vi "Calculations.vi"(0 "Trial in Progress IN":bool, 1 "DIO":bool[](array[boolean]), 2 "Trial Number":i16, 3 "cam_vel_ai_vlt":sgl[](array[numeric]), 5 "Sample Rate(s)":dbl=0.002 format="%.3f", 9 "Time Into Trial IN":dbl, 11 "Trial In Progress IN":T1, 12 "Inter-Trial Interval IN":bool) -> (4 "Data Cluster OUT":T2 {"Seconds Into Trial(s)" format="%#.10g"}, 6 "Trial Fraction of 1 Reached?":bool, 8 "Timeout Due to Mouse Not Moving?":bool, 10 "Wall MM Outputs":sgl[](array[numeric]), 14 "Trial Fraction OUT":dbl, 15 "Inter-Trial Interval Complete?":bool)   [LabVIEW 2018]
uses:
  controls/Data To Save.ctl
  controls/Trial Config Settings.ctl
  <vilib>/ptbypt/NI_PtbyPt.lvlib
  controls/RT_Cluster.ctl
panel:
  out "Speed_Time_Length":i32
  out "mean_lat_vel":dbl
  out "mean_for_vel":dbl
  out "Vball":dbl format="%.3f"
  out "lat_vel_array":dbl[](array[numeric])
  out "for_vel_array":dbl[](array[numeric])
  out "Cur_Speed_Ind":i32
  out "A_calib_matrix_row1":dbl[](array[numeric])
  out "A_calib_matrix_row0":dbl[](array[numeric])
  out "lat_ball_motion":dbl
  out "for_ball_motion":dbl
  out "zero_V":dbl[](array[numeric])
  out "step_V":dbl
  out "cam_vel_steps":dbl[](array[numeric])
  # "aClck_DI\nframe_clock_DO\nwhisker_video_ctrl_DO\nlick_signal_DI\nwater_valve_trigger\nlaser_ctrl\nleft_texture_ctrl_DO\nright_texture_ctrl_DO\ntrial_ephys_ctrl_DO\ntrial_iti_ctrl_DO\ntrial_on_ctrl_DO\nephys_clock_DO"
  # "*If Speed_Time_Length = 250\nthen averages are calculated every\n0.5 seconds since 1 data save takes\nplace every 0.002 seconds."
  # "="
  # "="
  # "avg"
  # "mean_for_vel"
  # "for_ball_motion (speed_time_length)"
  # "="
  # "="
  # "avg"
  # "mean_lat_vel"
  # "lat_ball_motion (speed_time_length)"
  # "cm/s"
  # "cm/s"
  # "2"
  # "2"
  # "="
  # "+"
  # "cm/s"
  # "for_ball_motion"
  # "lat_ball_motion"
  # "Left Wall"
  # "Vdc"
  # "Right Wall"
  # "Vdc"
  # "A_calib(0,0) x cam_vel_steps(0)"
  # "="
  # "A_calib(0,1) x cam_vel_steps(1)"
  # "sum"
  # "cm/s"
  # "A_calib(0,2) x cam_vel_steps(2)"
  # "A_calib(0,3) x cam_vel_steps(3)"
  # "A_calib(1,0) x cam_vel_steps(0)"
  # "="
  # "A_calib(1,1) x cam_vel_steps(1)"
  # "sum"
  # "cm/s"
  # "A_calib(1,2) x cam_vel_steps(2)"
  # "A_calib(1,3) x cam_vel_steps(3)"
  # "minus"
  # "="
  # "round"
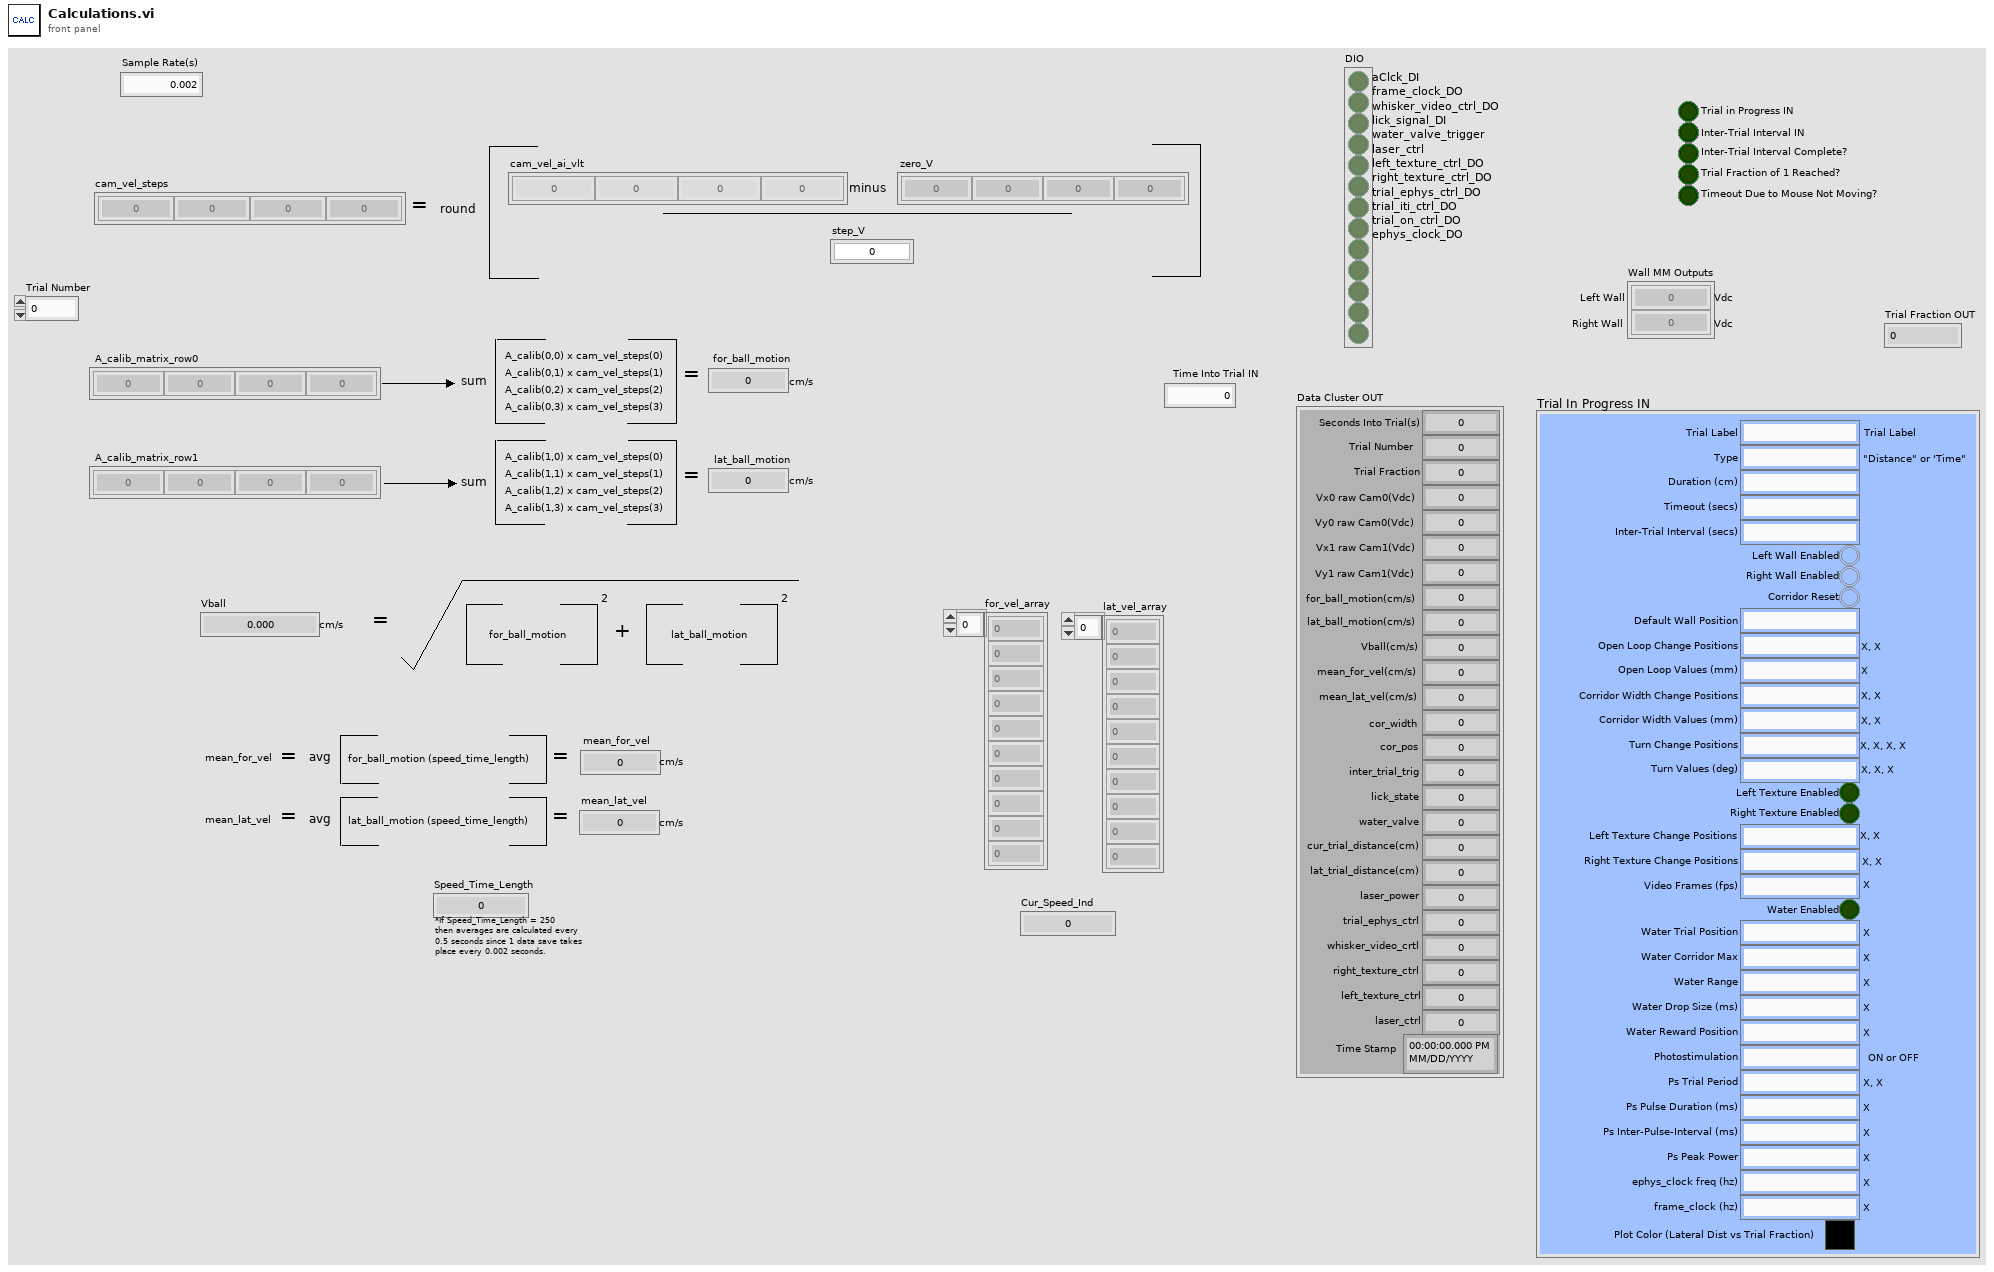
[diagram p1: front panel]
types:
  T1 = typedef "Trial Config Settings.ctl" = cluster{"Trial Label":string, "Type":string, "Timeout (secs)":string, "Inter-Trial Interval (secs)":string, "Left Wall Enabled":bool, "Right Wall Enabled":bool, "Corridor Reset":bool, "Default Wall Position":string, "Open Loop Change Positions":string, "Open Loop Values (mm)":string, "Corridor Width Change Positions":string, "Corridor Width Values (mm) ":string, "Turn Change Positions":string, "Turn Values (deg)":string, "Left Texture Change Positions":string, "Right Texture Change Positions":string, "Video Frames (fps)":string, "Water Enabled":bool, "Water Trial Position":string, "Photostimulation":string, "Water Corridor Max":string, "Water Range":string, "Water Drop Size (ms)":string, "Water Reward Position":string, "Duration (cm)":string, "Left Texture Enabled":bool, "Right Texture Enabled":bool, "Ps Trial Period":string, "Ps Inter-Pulse-Interval (ms)":string, "Ps Peak Power":string, "Ps Pulse Duration (ms)":string, "ephys_clock freq (hz)":string, "frame_clock (hz)":string, "Plot Color (Lateral Dist vs Trial Fraction)":u32}
  T2 = typedef "Data To Save.ctl" = cluster{"Vx0 raw Cam0(Vdc)":sgl, "Vy0 raw Cam0(Vdc)":sgl, "Vx1 raw Cam1(Vdc)":sgl, "Vy1 raw Cam1(Vdc)":sgl, "Seconds Into Trial(s)":dbl, "cor_width":sgl, "cor_pos":sgl, "for_ball_motion(cm/s)":sgl, "lat_ball_motion(cm/s)":sgl, "Vball(cm/s)":sgl, "mean_for_vel(cm/s)":sgl, "mean_lat_vel(cm/s)":sgl, "Trial Fraction":dbl, "Trial Number":i16, "inter_trial_trig":i16, "lick_state":i16, "water_valve":i16, "cur_trial_distance(cm)":dbl, "lat_trial_distance(cm)":dbl, "laser_power":dbl, "trial_ephys_ctrl":i16, "whisker_video_crtl":i16, "right_texture_ctrl":i16, "left_texture_ctrl":i16, "laser_ctrl":i16, "Time Stamp":timestamp}
  T3 = typedef "RT_Cluster.ctl" = cluster{"Data Cluster OUT":T2, "Corridor Reset":bool, "Wall Analog Outputs":sgl[], "Trial Fraction of 1 Reached?":bool, "Timeout Due to Mouse Not Moving?":bool, "Inter-Trial Interval Complete?":bool, "appended array":dbl[], "appended array 2":dbl[]}
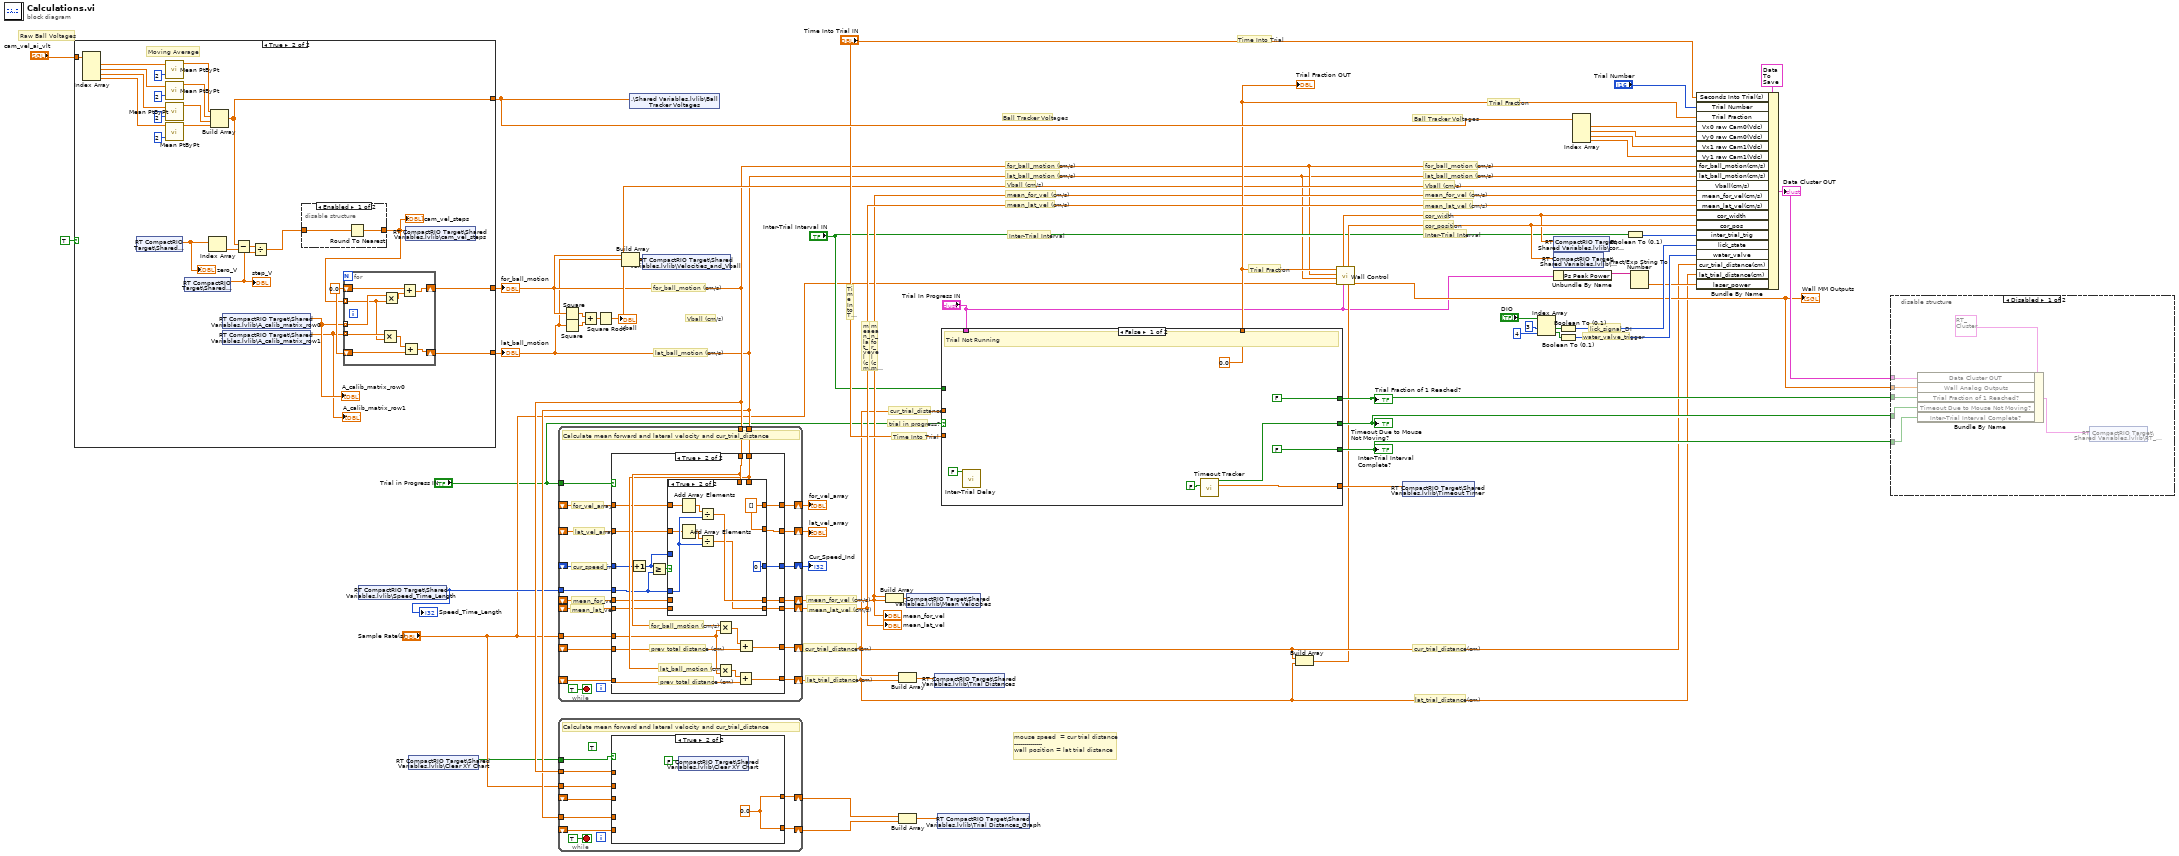
[diagram p0: block diagram]
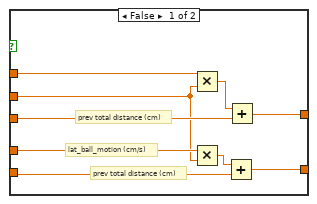
[diagram p3: hidden frame]
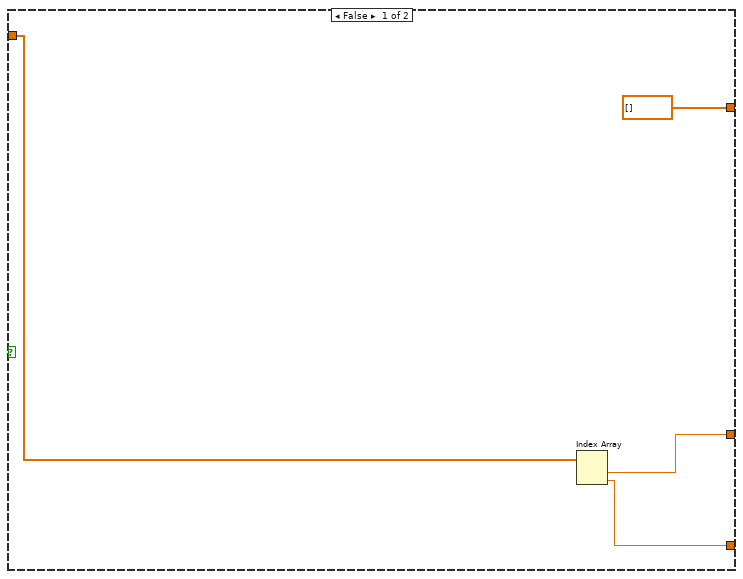
[diagram p4: hidden frame]
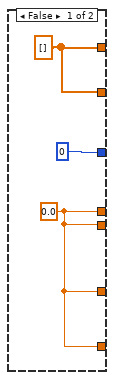
[diagram p6: hidden frame]
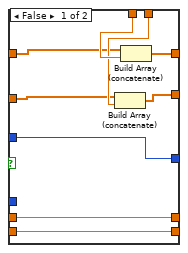
[diagram p7: hidden frame]
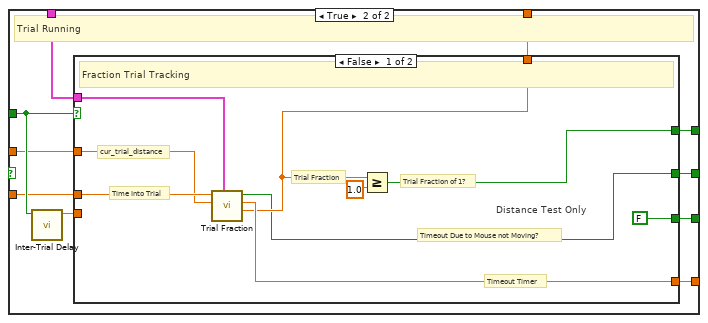
[diagram p8: hidden frame]
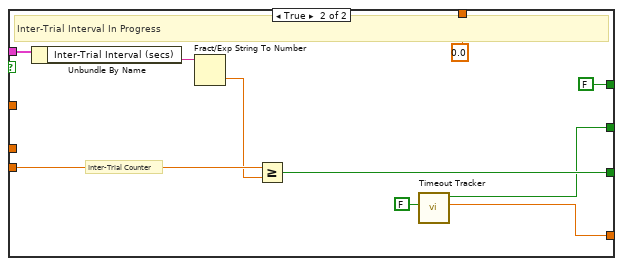
[diagram p9: hidden frame]
diagram:
  # "mouse speed  = cur trial distance\n--------------\nwall position = lat trial distance"
  # "Trial Fraction"
  # "lat_trial_distance(cm)"
  # "mean_for_vel (cm/s)"
  # "mean_lat_vel (cm/s)"
  # "cur_trial_distance(cm)"
  # "trial in progress?"
  # "for_ball_motion (cm/s)"
  # "lat_ball_motion (cm/s)"
  # "mean_lat_vel (cm/s)"
  # "mean_for_vel (cm/s)"
  # "Vball (cm/s)"
  # "lat_trial_distance(cm)"
  # "Inter-Trial Interval"
  # "cur_trial_distance(cm)"
  # "mean_for_vel (cm/s)"
  # "mean_lat_vel (cm/s)"
  # "Time Into Trial"
  # "Time Into Trial"
  # "cur_trial_distance"
  # "Vball (cm/s)"
  # "for_ball_motion (cm/s)"
  # "lat_ball_motion (cm/s)"
  # "Inter-Trial Interval"
  # "cor_position"
  # "cor_width"
  # "Ball Tracker Voltages"
  # "Time Into Trial"
  # "Ball Tracker Voltages"
  # "for_ball_motion (cm/s)"
  # "lat_ball_motion (cm/s)"
  # "mean_lat_vel (cm/s)"
  # "mean_for_vel (cm/s)"
  # "Vball (cm/s)"
  # "Trial Fraction"
  # "water_valve_trigger"
  # "lick_signal_DI"
  # "Raw Ball Voltages"
  n1 = case shown="True" TRUE {
    tunnel: "cam_vel_ai_vlt" -> [w59 w69]
    tunnel: [dbl[] [] w64] -> w48
    tunnel: [w58 w61] -> w13
    tunnel: [w57 w60] -> w12
    frame False {
      n2 = Index Array(array=w59) -> (element #1=w58:sgl, element #2=w57:sgl)  [unwired: 2 in]
    }
    frame True {
      w84 = 0.0
      # "Moving Average"
      n3 = Index Array(array=w69) -> (element #1=w68:sgl, element #2=w67:sgl, element #3=w66:sgl, element #4=w65:sgl)  [unwired: 4 in]
      n4 = shared-variable "RT CompactRIO Target\\Shared Variables.lvlib\\zero_V"() -> (w80:dbl[])  [unwired: 1 in, 1 out]
      "zero_V" <- w80
      n5 = call <vilib>:"Mean PtByPt.vi"("x"=w68, "sample length"=2) -> ("mean"=w63:dbl)  [unwired: 2 in, 1 out]
      n6 = call <vilib>:"Mean PtByPt.vi"("x"=w67, "sample length"=2) -> ("mean"=w72:dbl)  [unwired: 2 in, 1 out]
      n7 = call <vilib>:"Mean PtByPt.vi"("x"=w66, "sample length"=2) -> ("mean"=w71:dbl)  [unwired: 2 in, 1 out]
      n8 = call <vilib>:"Mean PtByPt.vi"("x"=w65, "sample length"=2) -> ("mean"=w70:dbl)  [unwired: 2 in, 1 out]
      n9 = shared-variable "RT CompactRIO Target\\Shared Variables.lvlib\\step_V"() -> (w79:dbl)  [unwired: 1 in, 1 out]
      "step_V" <- w79
      n10 = Index Array(array=w80) -> (element=w82:dbl)  [unwired: 1 in]
      n11 = Build Array(w63, w72, w71, w70) -> (w64:dbl[])
      n12 = shared-variable "RT CompactRIO Target\\Shared Variables.lvlib\\A_calib_matrix_row0"() -> (w78:dbl[])  [unwired: 1 in, 1 out]
      "A_calib_matrix_row0" <- w78
      n13 = shared-variable "RT CompactRIO Target\\Shared Variables.lvlib\\A_calib_matrix_row1"() -> (w77:dbl[])  [unwired: 1 in, 1 out]
      "A_calib_matrix_row1" <- w77
      n14 = Subtract ("Subtract.vi")(x=w64, y=w82) -> (x-y=w83:dbl[])
      n15 = Divide(x=w83, y=w79) -> (x/y=w81:dbl[])
      n16 = disable-structure shown="Enabled" {
        disable-tunnel: w81 -> [w86 w87]
        disable-tunnel: [w85 w87] -> w62
        frame Enabled {
          n17 = Round To Nearest(number=w86) -> (nearest integer value=w85:dbl[])
        }
        frame Disabled {
        }
      }
      "cam_vel_steps" <- w62
      n18 = for {
        tunnel: w78 -> [w96] mode=indexing
        tunnel: w77 -> [w95] mode=indexing
        tunnel: w62 -> [w94] mode=indexing
        shift-right: [w91] -> w61
        shift-left: w84 -> [w92]
        shift-right: [w90] -> w60
        shift-left: w84 -> [w88]
        n19 = Multiply(x=w95, y=w94) -> (x*y=w89:dbl)
        n20 = Multiply(x=w96, y=w94) -> (x*y=w93:dbl)
        n21 = Add(x=w92, y=w93) -> (x+y=w91:dbl)
        n22 = Add(x=w89, y=w88) -> (x+y=w90:dbl)
      }
      n23 = shared-variable "RT CompactRIO Target\\Shared Variables.lvlib\\cam_vel_steps"(w62) -> ()  [unwired: 1 in, 1 out]
    }
  }
  "for_ball_motion" <- w13
  "lat_ball_motion" <- w12
  n24 = shared-variable "RT CompactRIO Target\\Shared Variables.lvlib\\Speed_Time_Length"() -> (w11:i32)  [unwired: 1 in, 1 out]
  "Speed_Time_Length" <- w11
  n25 = shared-variable "RT CompactRIO Target\\Shared Variables.lvlib\\Clear XY Chart"() -> (w2:bool)  [unwired: 1 in, 1 out]
  n26 = while {
    tunnel: w13 -> [w116]
    tunnel: w12 -> [w115]
    shift-right: [w114] -> w25
    shift-left: _ -> [w111]
    shift-right: [w113] -> w24
    shift-left: _ -> [w110]
    shift-right: [w108] -> w23
    shift-left: _ -> [w109]
    shift-right: [w106] -> w50
    shift-left: _ -> [w104]
    shift-right: [w107] -> w28
    shift-left: _ -> [w105]
    tunnel: w11 -> [w103]
    tunnel: "Trial in Progress IN" -> [w98]
    shift-right: [w102] -> w6
    shift-left: _ -> [w101]
    shift-right: [w100] -> w5
    shift-left: _ -> [w99]
    tunnel: "Sample Rate(s)" -> [w97]
    stop <- TRUE stop-if-true
    # "mean_for_vel"
    # "mean_lat_vel"
    # "cur_speed_ind"
    # "lat_vel_array"
    # "for_vel_array"
    # "Calculate mean forward and lateral velocity and cur_trial_distance"
    n27 = case shown="True" w98 {
      tunnel: w116 -> [_ w141]
      tunnel: w115 -> [_ w140]
      tunnel: [w119 w139] -> w114
      tunnel: [w119 w138] -> w113
      tunnel: w111 -> [_ w137]
      tunnel: w110 -> [_ w136]
      tunnel: w109 -> [_ w135]
      tunnel: [0 w134] -> w108
      tunnel: [w117 w133] -> w107
      tunnel: [w117 w132] -> w106
      tunnel: w105 -> [_ w131]
      tunnel: w104 -> [_ w130]
      tunnel: w103 -> [_ w129]
      tunnel: [w117 w128] -> w102
      tunnel: w101 -> [_ w127]
      tunnel: [w117 w126] -> w100
      tunnel: w99 -> [_ w125]
      tunnel: w97 -> [_ w120]
      frame False {
        w119 = dbl[] []
        w117 = 0.0 ("mean_for_vel")
      }
      frame True {
        # "prev total distance (cm)"
        # "lat_ball_motion (cm/s)"
        # "prev total distance (cm)"
        # "for_ball_motion (cm/s)"
        n28 = Increment(x=w135) -> (x+1=w123:i32)
        n29 = Greater Or Equal?(x=w123, y=w129) -> (x >= y?=w124:bool)
        n30 = case shown="True" w124 {
          tunnel: [w149 w159] -> w139
          tunnel: [w147 w159] -> w138
          tunnel: w129 -> [_ w156]
          tunnel: w141 -> [w150 _]
          tunnel: w140 -> [w148 _]
          tunnel: w137 -> [w146 w155]
          tunnel: w136 -> [w145 w154]
          tunnel: [w144 0] -> w134
          tunnel: w123 -> [w144 _]
          tunnel: [w143 w152] -> w133
          tunnel: [w142 w151] -> w132
          tunnel: w131 -> [w143 _]
          tunnel: w130 -> [w142 _]
          frame False {
            n31 = Build Array (concatenate)(w145, w148) -> (w147:dbl[])
            n32 = Build Array (concatenate)(w146, w150) -> (w149:dbl[])
          }
          frame True {
            w159 = dbl[] []
            n33 = Add Array Elements(numeric array=w155) -> (sum=w158:dbl)
            n34 = Add Array Elements(numeric array=w154) -> (sum=w157:dbl)
            n35 = Divide(x=w158, y=w156) -> (x/y=w152:dbl)
            n36 = Divide(x=w157, y=w156) -> (x/y=w151:dbl)
          }
        }
        n37 = Multiply(x=w141, y=w120) -> (x*y=w122:dbl)
        n38 = Multiply(x=w140, y=w120) -> (x*y=w121:dbl)
        n39 = Add(x=w121, y=w125) -> (x+y=w126:dbl)
        n40 = Add(x=w122, y=w127) -> (x+y=w128:dbl)
      }
    }
  }
  "mean_for_vel" <- w28
  "mean_lat_vel" <- w50
  "for_vel_array" <- w25
  "lat_vel_array" <- w24
  "Cur_Speed_Ind" <- w23
  n41 = while {
    tunnel: w13 -> [w168]
    tunnel: w12 -> [w167]
    shift-right: [w165] -> w8
    shift-left: _ -> [w164]
    shift-right: [w163] -> w9
    shift-left: _ -> [w162]
    tunnel: "Sample Rate(s)" -> [w161]
    tunnel: w2 -> [w160]
    stop <- TRUE stop-if-true
    (unwired) TRUE
    # "Calculate mean forward and lateral velocity and cur_trial_distance"
    n42 = case shown="True" w160 {
      tunnel: w168 -> [w177 _]
      tunnel: w167 -> [w176 _]
      tunnel: [w175 w179] -> w165
      tunnel: w164 -> [w174 _]
      tunnel: [w173 w179] -> w163
      tunnel: w162 -> [w172 _]
      tunnel: w161 -> [w169 _]
      frame False {
        # "prev total distance (cm)"
        # "lat_ball_motion (cm/s)"
        # "prev total distance (cm)"
        n43 = Multiply(x=w177, y=w169) -> (x*y=w171:dbl)
        n44 = Multiply(x=w176, y=w169) -> (x*y=w170:dbl)
        n45 = Add(x=w170, y=w172) -> (x+y=w173:dbl)
        n46 = Add(x=w171, y=w174) -> (x+y=w175:dbl)
      }
      frame True {
        w179 = 0.0 ("mean_for_vel")
        n47 = shared-variable "RT CompactRIO Target\\Shared Variables.lvlib\\Clear XY Chart"(FALSE ("Clear XY Chart")) -> ()  [unwired: 1 in, 1 out]
      }
    }
  }
  n48 = Square(x=w13) -> (x^2=w31:dbl)
  n49 = Square(x=w12) -> (x^2=w30:dbl)
  n50 = Add(x=w31, y=w30) -> (x+y=w29:dbl)
  n51 = Square Root(x=w29) -> (sqrt(x)=w22:dbl)
  "Vball" <- w22
  n52 = Build Array(w13, w12, w22) -> (w54:dbl[])
  n53 = shared-variable ".\\Shared Variables.lvlib\\Ball Tracker Voltages"(w48) -> ()  [unwired: 1 in, 1 out]
  n54 = shared-variable "RT CompactRIO Target\\Shared Variables.lvlib\\Velocities_and_Vball"(w54) -> ()  [unwired: 1 in, 1 out]
  n55 = Build Array(w28, w28) -> (w55:dbl[])
  n56 = Build Array(w6, w5) -> (w21:dbl[])
  n57 = Build Array(w8, w9) -> (w7:dbl[])
  n58 = shared-variable "RT CompactRIO Target\\Shared Variables.lvlib\\Mean Velocities"(w55) -> ()  [unwired: 1 in, 1 out]
  n59 = shared-variable "RT CompactRIO Target\\Shared Variables.lvlib\\Trial Distances"(w21) -> ()  [unwired: 1 in, 1 out]
  n60 = shared-variable "RT CompactRIO Target\\Shared Variables.lvlib\\Trial Distances_Graph"(w7) -> ()  [unwired: 1 in, 1 out]
  n61 = case shown="False" "Trial in Progress IN" {
    tunnel: "Inter-Trial Interval IN" -> [_ w195]
    tunnel: "Trial In Progress IN" -> [_ w194]
    tunnel: "Time Into Trial IN" -> [_ w193]
    tunnel: w6 -> [_ w192]
    tunnel: [w185 w191] -> w34
    tunnel: [FALSE w190] -> w17
    tunnel: [FALSE w189] -> w19
    tunnel: [0.0 ("Trial Fraction") w188] -> w35
    tunnel: [w180 w187] -> w18
    frame False {
      # "Trial Not Running"
      n62 = call "Inter-Trial Delay.vi"("Start Inter-Trial Delay?"=FALSE) -> ()  [unwired: 10 in, 1 out]
      n63 = call "Timeout Tracker.vi"("Mouse Not Moving?"=FALSE) -> ("Timeout Timer"=w185:dbl, "Timeout"=w180:bool)  [unwired: 9 in]
    }
    frame True {
      # "Trial Running"
      n64 = call "Inter-Trial Delay.vi"("Start Inter-Trial Delay?"=w195) -> ("Inter-Trial Counter (secs)"=w196:dbl)  [unwired: 10 in]
      n65 = case shown="False" w195 {
        tunnel: [w202 w214] -> w191
        tunnel: w196 -> [_ w213]
        tunnel: w194 -> [w204 w212]
        tunnel: w193 -> [w203 _]
        tunnel: w192 -> [w197 _]
        tunnel: [FALSE w209] -> w190
        tunnel: [w199 FALSE] -> w189
        tunnel: [w200 0.0 ("Trial Fraction")] -> w188
        tunnel: [w198 w206] -> w187
        frame False {
          # "cur_trial_distance"
          # "Timeout Timer"
          # "Distance Test Only"
          # "Timeout Due to Mouse not Moving?"
          # "Time Into Trial"
          # "Trial Fraction of 1?"
          # "Trial Fraction"
          # "Fraction Trial Tracking"
          n66 = call "Trial Fraction.vi"("Trial In Progress IN"=w204, "cur_trial_dist"=w197, "Time into Trial"=w203) -> ("Trial Fraction"=w200:dbl, "Timeout Timer"=w202:dbl, "Timeout?"=w198:bool)  [unwired: 6 in]
          n67 = Greater Or Equal?(x=w200, y=1.0) -> (x >= y?=w199:bool)
        }
        frame True {
          # "Inter-Trial Counter"
          # "Inter-Trial Interval In Progress"
          n68 = Unbundle By Name(w212) -> ("Inter-Trial Interval (secs)"=w211:string)
          n69 = Fract/Exp String To Number(string=w211) -> (number=w210:dbl)  [unwired: 3 in, 1 out]
          n70 = Greater Or Equal?(x=w213, y=w210) -> (x >= y?=w209:bool)
          n71 = call "Timeout Tracker.vi"("Mouse Not Moving?"=FALSE) -> ("Timeout Timer"=w214:dbl, "Timeout"=w206:bool)  [unwired: 9 in]
        }
      }
    }
  }
  "Inter-Trial Interval Complete?" <- w17
  "Trial Fraction of 1 Reached?" <- w19
  "Trial Fraction OUT" <- w35
  "Timeout Due to Mouse Not Moving?" <- w18
  n72 = Build Array(w6, w5) -> (w4:dbl[])
  n73 = call "Wall Control.vi"("Trial Distances"=w4, "Trial In Progress IN"="Trial In Progress IN", "Sample Rate(s)"="Sample Rate(s)", "lat_ball_motion IN"=w12, "for_ball_motion IN"=w13, "Trial Fraction IN"=w35) -> ("Wall MM Outputs"=w15:dbl[], "cor_pos OUT"=w33:dbl, "cor_width OUT"=w32:dbl)  [unwired: 3 in]
  "Wall MM Outputs" <- w15
  n74 = shared-variable "RT CompactRIO Target\\Shared Variables.lvlib\\Timeout Timer"(w34) -> ()  [unwired: 1 in, 1 out]
  n75 = Index Array(array="DIO", index #1=3 ("index"), index #2=4 ("index")) -> (element #1=w43:bool, element #2=w38:bool)
  n76 = shared-variable "RT CompactRIO Target\\Shared Variables.lvlib\\cor_width"(w32) -> ()  [unwired: 1 in, 1 out]
  n77 = shared-variable "RT CompactRIO Target\\Shared Variables.lvlib\\cor_pos"(w33) -> ()  [unwired: 1 in, 1 out]
  n78 = Unbundle By Name("Trial In Progress IN") -> ("Ps Peak Power"=w27:string)
  n79 = Boolean To (0,1)(Boolean=w43) -> (0, 1=w42:i16)
  n80 = Boolean To (0,1)(Boolean=w38) -> (0, 1=w37:i16)
  n81 = Index Array(array=w48) -> (element #1=w46:dbl, element #2=w47:dbl, element #3=w52:dbl, element #4=w51:dbl)  [unwired: 4 in]
  n82 = Boolean To (0,1)(Boolean="Inter-Trial Interval IN") -> (0, 1=w40:i16)
  n83 = Fract/Exp String To Number(string=w27) -> (number=w26:dbl)  [unwired: 3 in, 1 out]
  n84 = Bundle By Name(cluster=T2 {"Vx0 raw Cam0(Vdc)"=0.0, "Vy0 raw Cam0(Vdc)"=0.0, "Vx1 raw Cam1(Vdc)"=0.0, "Vy1 raw Cam1(Vdc)"=0.0, "Seconds Into Trial(s)"=0.0, "cor_width"=0.0, "cor_pos"=0.0, "for_ball_motion(cm/s)"=0.0, "lat_ball_motion(cm/s)"=0.0, "Vball(cm/s)"=0.0, "mean_for_vel(cm/s)"=0.0, "mean_lat_vel(cm/s)"=0.0, "Trial Fraction"=0.0, "Trial Number"=0, "inter_trial_trig"=0, "lick_state"=0, "water_valve"=0, "cur_trial_distance(cm)"=0.0, "lat_trial_distance(cm)"=0.0, "laser_power"=0.0, "trial_ephys_ctrl"=0, "whisker_video_crtl"=0, "right_texture_ctrl"=0, "left_texture_ctrl"=0, "laser_ctrl"=0, "Time Stamp"=timestamp(0 s since 1904-01-01)} ("Data"), "Seconds Into Trial(s)"="Time Into Trial IN", "Trial Number"="Trial Number", "Trial Fraction"=w35, "Vx0 raw Cam0(Vdc)"=w46, "Vy0 raw Cam0(Vdc)"=w47, "Vx1 raw Cam1(Vdc)"=w52, "Vy1 raw Cam1(Vdc)"=w51, "for_ball_motion(cm/s)"=w13, "lat_ball_motion(cm/s)"=w12, "Vball(cm/s)"=w22, "mean_for_vel(cm/s)"=w28, "mean_lat_vel(cm/s)"=w50, "cor_width"=w32, "cor_pos"=w33, "inter_trial_trig"=w40, "lick_state"=w42, "water_valve"=w37, "cur_trial_distance(cm)"=w6, "lat_trial_distance(cm)"=w5, "laser_power"=w26) -> (w20:T2)
  "Data Cluster OUT" <- w20
  n85 = disable-structure shown="Disabled" {
    disable-tunnel: w20 -> [w221 _]
    disable-tunnel: w19 -> [w220 _]
    disable-tunnel: w18 -> [w219 _]
    disable-tunnel: w17 -> [w218 _]
    disable-tunnel: w15 -> [w216 _]
    frame Disabled {
      n86 = Bundle By Name(cluster=T3 {"Data Cluster OUT"={"Vx0 raw Cam0(Vdc)"=0.0, "Vy0 raw Cam0(Vdc)"=0.0, "Vx1 raw Cam1(Vdc)"=0.0, "Vy1 raw Cam1(Vdc)"=0.0, "Seconds Into Trial(s)"=0.0, "cor_width"=0.0, "cor_pos"=0.0, "for_ball_motion(cm/s)"=0.0, "lat_ball_motion(cm/s)"=0.0, "Vball(cm/s)"=0.0, "mean_for_vel(cm/s)"=0.0, "mean_lat_vel(cm/s)"=0.0, "Trial Fraction"=0.0, "Trial Number"=0, "inter_trial_trig"=0, "lick_state"=0, "water_valve"=0, "cur_trial_distance(cm)"=0.0, "lat_trial_distance(cm)"=0.0, "laser_power"=0.0, "trial_ephys_ctrl"=0, "whisker_video_crtl"=0, "right_texture_ctrl"=0, "left_texture_ctrl"=0, "laser_ctrl"=0, "Time Stamp"=timestamp(0 s since 1904-01-01)}, "Corridor Reset"=FALSE, "Wall Analog Outputs"=[], "Trial Fraction of 1 Reached?"=FALSE, "Timeout Due to Mouse Not Moving?"=FALSE, "Inter-Trial Interval Complete?"=FALSE, "appended array"=[], "appended array 2"=[]}, "Data Cluster OUT"=w221, "Wall Analog Outputs"=w216, "Trial Fraction of 1 Reached?"=w220, "Timeout Due to Mouse Not Moving?"=w219, "Inter-Trial Interval Complete?"=w218) -> (w217:T3)
      n87 = shared-variable "RT CompactRIO Target\\Shared Variables.lvlib\\RT_Cluster"(w217) -> ()  [unwired: 1 in, 1 out]
    }
    frame Enabled {
    }
  }
